vi "Set Data Value.vi"(8 "error in (no error)":errorcluster, 9 "Data":string, 11 "stringPayload in":refnum<class "stringPayload.lvclass">) -> (0 "error out":errorcluster, 3 "stringPayload out":refnum<class "stringPayload.lvclass">)   [LabVIEW 2017, in "messagesPayload.lvlib" / "stringPayload.lvclass"]
uses:
  stringPayload.lvclass
  stringPayload.lvclass/stringPayload.ctl
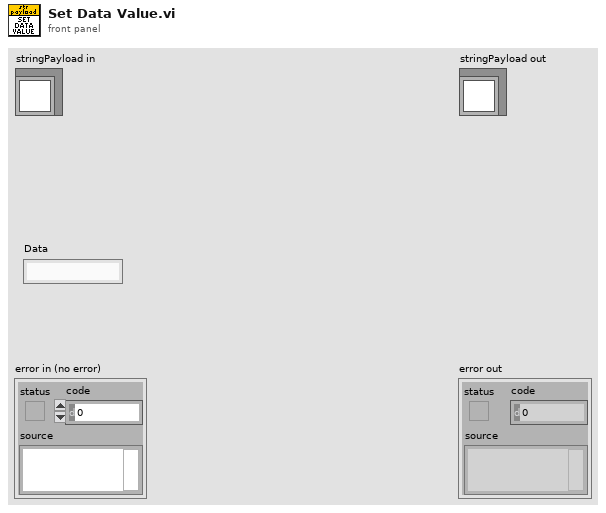
[diagram p1: front panel]
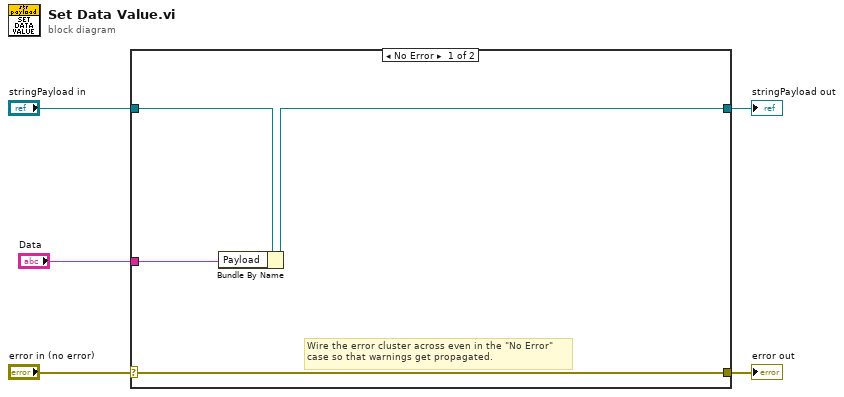
[diagram p0: block diagram]
diagram:
  n1 = case shown="No Error" "error in (no error)" {
    selector: "error in (no error)" -> [w8 w11]
    tunnel: [w8 w11] -> w4
    tunnel: [w7 w10] -> w2
    tunnel: "stringPayload in" -> [w9 w10]
    tunnel: "Data" -> [w6 _]
    frame No Error {
      # "Wire the error cluster across even in the \"No Error\"\ncase so that warnings get propagated."
      n2 = Bundle By Name(cluster=w9, "Payload"=w6) -> (w7:refnum<class "stringPayload.lvclass">)
    }
    frame Error {
    }
  }
  "error out" <- w4
  "stringPayload out" <- w2
